vi "vision2.vi"(8 "error in":errorcluster) -> (0 "error out":errorcluster)   [LabVIEW 2017]
uses:
  <vilib>/userdefined/High Color/IMAQdx.ctl
  <vilib>/vision/driver/NI_Vision_Acquisition_Software.lvlib
panel:
  out "Edges Coordinates (Edge Detector 1)":cluster{"X":sgl, "Y":sgl}[](array[cluster]) {"Y" format="%.2f"; "X" format="%.2f"}
  out "Image":T1(plugin-control)
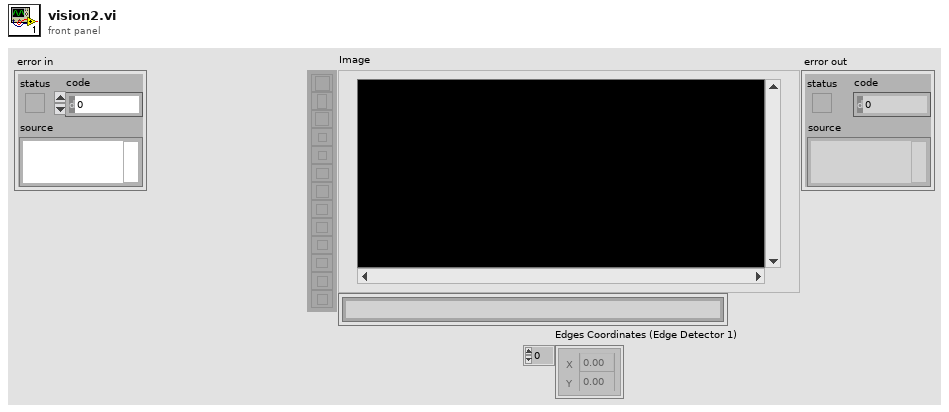
[diagram p1: front panel]
types:
  T1 = typedef "IMAQ Image.ctl" = refnum<image>
  T2 = typedef "IMAQdx.ctl" = refnum<k21>
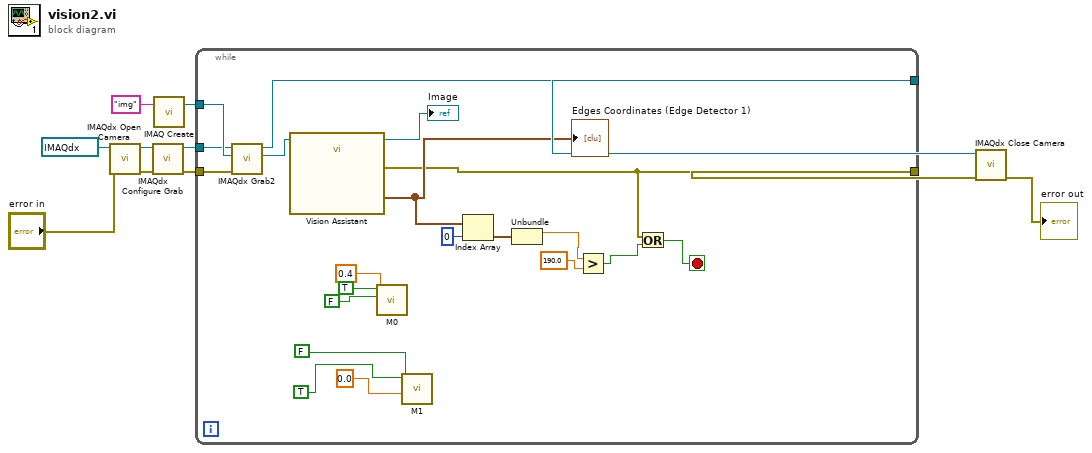
[diagram p0: block diagram]
diagram:
  n1 = call <vilib>:"IMAQdx Open Camera.vi"("error in"="error in", "Session In"=T2 "cam1") -> ("error out"=w5:errorcluster, "Session Out"=w8:T2)  [unwired: 8 in]
  n2 = call <vilib>:"IMAQdx Configure Grab.vi"("error in"=w5, "Session In"=w8) -> ("error out"=w6:errorcluster, "Session Out"=w9:T2)  [unwired: 8 in]
  n3 = call "IMAQ Create"("Image Name"="img") -> ("New Image"=w7:T1)  [unwired: 4 in, 1 out]
  n4 = while {
    tunnel: w6 -> [w31]
    tunnel: w7 -> [w30]
    tunnel: w9 -> [w29]
    tunnel: [w28] -> w10
    tunnel: [w21] -> w11
    stop <- w22 stop-if-true
    n5 = call <vilib>:"IMAQdx Grab2.vi"("error in"=w31, "Image In"=w30, "Session In"=w29) -> ("Image Out"=w26:T1, "Session Out"=w28:T2)  [unwired: 5 in, 2 out]
    n6 = call "Vision Assistant"("Image In"=w26) -> ("Image Out"=→"Image":T1, "Edges Coordinates (Edge Detector 1)"=w25:cluster{"X":sgl, "Y":sgl}[], "error out"=w21:errorcluster)  [unwired: 24 in]
    "Edges Coordinates (Edge Detector 1)" <- w25
    n7 = call "M0.vi"("Duty Cycle"=0.4, "назад"=FALSE ("вперед"), "вперед"=TRUE ("назад")) -> ()  [unwired: 8 in, 1 out]
    n8 = call "M1.vi"("Duty Cycle"=0.0, "назад"=FALSE ("вперед"), "вперед"=TRUE ("назад")) -> ()  [unwired: 8 in, 1 out]
    n9 = Index Array(array=w25, index=0) -> (element=w23:cluster{"X":sgl, "Y":sgl})
    n10 = Unbundle(w23) -> ("X"=w13:sgl)  [unwired: 1 out]
    n11 = Greater?(x=w13, y=sgl 190.0) -> (0:w12:bool)
    n12 = Or(x=w21, y=w12) -> (x .or. y?=w22:bool)
  }
  n13 = call <vilib>:"IMAQdx Close Camera.vi"("error in"=w11, "Session In"=w10) -> ("error out"=→"error out":errorcluster)  [unwired: 9 in]
